vi "QPSK_awgn.vi"(8 "error in":errorcluster, 9 "snr":dbl, 10 "txSig":cdb[](array[numeric]), 11 "Path In":path) -> (0 "error out":errorcluster, 2 "rxSig":cdb[](array[numeric]), 3 "Path Out":path)   [LabVIEW 2015]
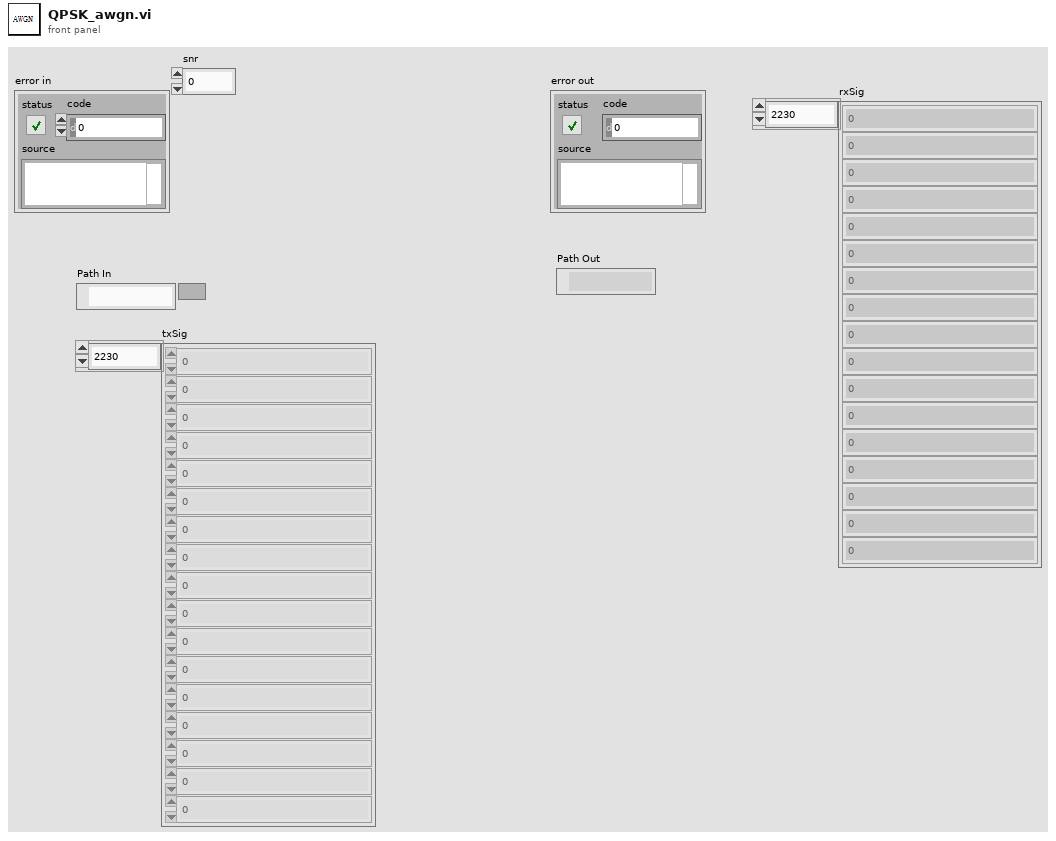
[diagram p1: front panel]
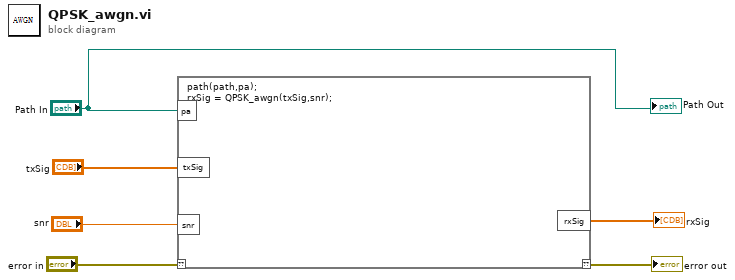
[diagram p0: block diagram]
diagram:
  n1 = script code="path(path,pa);\nrxSig = QPSK_awgn(txSig,snr);"("??"="error in", "pa"="Path In", "txSig"="txSig", "snr"="snr") -> ("??"=→"error out":errorcluster, "rxSig"=→"rxSig":cdb[])
  "Path Out" <- "Path In"
